vi "ObstacleEnemyRadius.vi"(4 "Goal":dbl[](array[numeric]), 6 "Initial State":dbl[](array[numeric]), 9 "Robot enemy":T1={"id"=0, "function"=enum."Attacker", "x"=0.0, "y"=0.0, "orientation"=0.0, "v_tangent"=0.0, "v_normal"=0.0, "v_ang"=0.0, "kick_x"=0.0, "kick_z"=0.0, "dribble"=FALSE, "Timestamp"=timestamp(0 s since 1904-01-01), "estimatives"={"est_v_tangent"=0.0, "est_v_normal"=0.0, "est_vx"=0.0, "est_vy"=0.0, "Pos Robot Est"=[]}, "dest_x_kick"=0.0, "dest_y_kick"=0.0, "Gap Coord"=[], "States"=enum."GoToTangent", "Path "=[], "Path  Smooth"=[], "Dest"=[]}, 10 "Robot in":T1={"id"=0, "function"=enum."Attacker", "x"=0.0, "y"=0.0, "orientation"=0.0, "v_tangent"=0.0, "v_normal"=0.0, "v_ang"=0.0, "kick_x"=0.0, "kick_z"=0.0, "dribble"=FALSE, "Timestamp"=timestamp(0 s since 1904-01-01), "estimatives"={"est_v_tangent"=0.0, "est_v_normal"=0.0, "est_vx"=0.0, "est_vy"=0.0, "Pos Robot Est"=[]}, "dest_x_kick"=0.0, "dest_y_kick"=0.0, "Gap Coord"=[], "States"=enum."GoToTangent", "Path "=[], "Path  Smooth"=[], "Dest"=[]}) -> (2 "obstacle enemy radius":dbl)   [LabVIEW 2017]
uses:
  Core/AI Robot.ctl
  Intel/Functions Enum.ctl
  Intel/AttackerStates.ctl
  PathDests.ctl
  PathDest.ctl
  <vilib>/Analysis/_algsub.llb/Real Vector Norm.vi
  <vilib>/Analysis/NI_AALPro.lvlib
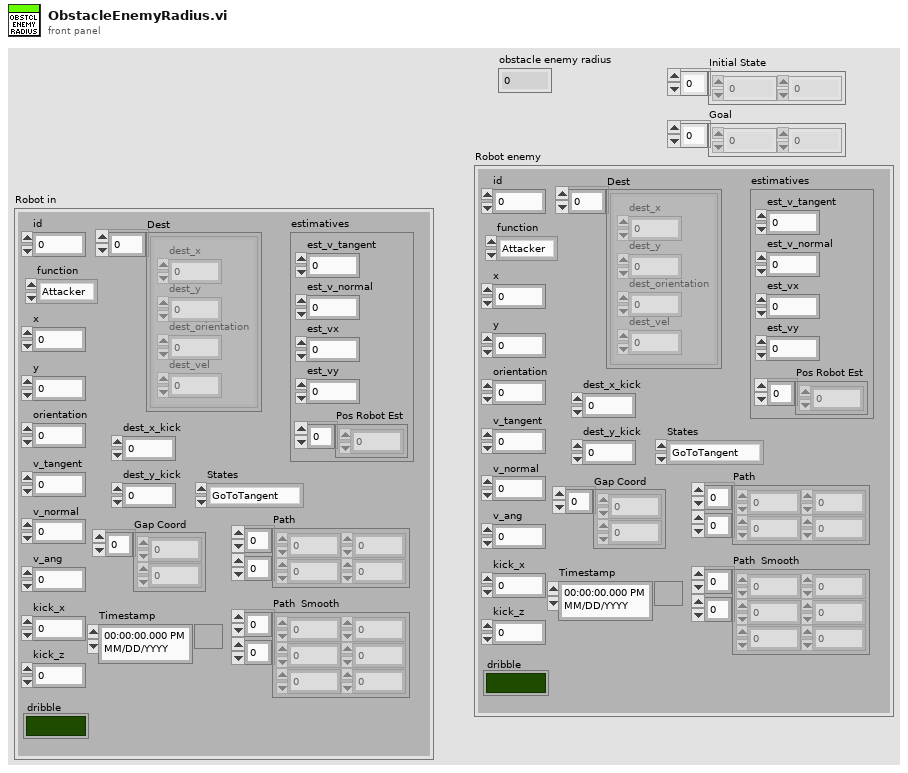
[diagram p1: front panel]
types:
  T1 = typedef "AI Robot.ctl" = cluster{"id":u32, "function":T2, "x":dbl, "y":dbl, "orientation":dbl, "v_tangent":dbl, "v_normal":dbl, "v_ang":dbl, "kick_x":dbl, "kick_z":dbl, "dribble":bool, "Timestamp":timestamp, "estimatives":cluster{"est_v_tangent":dbl, "est_v_normal":dbl, "est_vx":dbl, "est_vy":dbl, "Pos Robot Est":dbl[]}, "dest_x_kick":dbl, "dest_y_kick":dbl, "Gap Coord":dbl[], "States":T3, "Path ":dbl[][], "Path  Smooth":dbl[][], "Dest":T4}
  T2 = typedef "Functions Enum.ctl" = enum16{"Attacker", "Goalie", "Defender", "Striker", "Goto 0", "Dummy", "Kicker", "ZigZag"}
  T3 = typedef "AttackerStates.ctl" = enum16{"Pass", "GoToTangent", "BallGetting", "GoToKick", ""}
  T4 = typedef "PathDests.ctl" = T5[]
  T5 = typedef "PathDest.ctl" = cluster{"dest_x":dbl, "dest_y":dbl, "dest_orientation":dbl, "dest_vel":dbl}
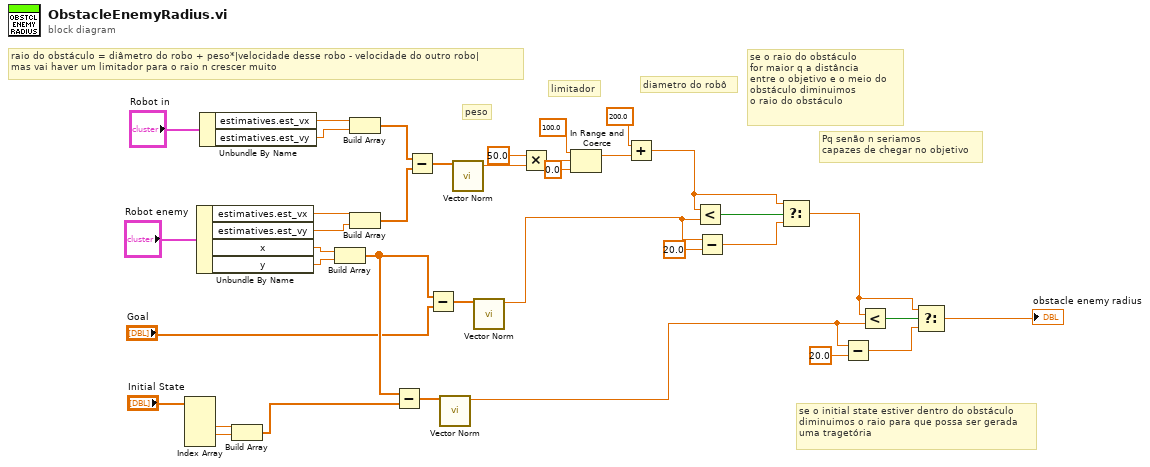
[diagram p0: block diagram]
diagram:
  # "se o initial state estiver dentro do obstáculo\ndiminuimos o raio para que possa ser gerada\numa tragetória"
  # "limitador"
  # "peso"
  # "diametro do robô"
  # "Pq senão n seriamos\ncapazes de chegar no objetivo"
  # "se o raio do obstáculo\nfor maior q a distância \nentre o objetivo e o meio do \nobstáculo diminuimos \no raio do obstáculo"
  # "raio do obstáculo = diâmetro do robo + peso*|velocidade desse robo - velocidade do outro robo|\nmas vai haver um limitador para o raio n crescer muito"
  n1 = Index Array(array="Initial State") -> (element #2=w3:dbl, element #3=w2:dbl)  [unwired: 4 in, 2 out]
  n2 = Unbundle By Name("Robot enemy") -> ("estimatives.est_vx"=w35:dbl, "estimatives.est_vy"=w34:dbl, "x"=w21:dbl, "y"=w20:dbl)
  n3 = Unbundle By Name("Robot in") -> ("estimatives.est_vx"=w33:dbl, "estimatives.est_vy"=w32:dbl)
  n4 = Build Array(w3, w2) -> (w1:dbl[])
  n5 = Build Array(w21, w20) -> (w12:dbl[])
  n6 = Build Array(w33, w32) -> (w31:dbl[])
  n7 = Build Array(w35, w34) -> (w30:dbl[])
  n8 = Subtract(x=w12, y=w1) -> (x-y=w13:dbl[])
  n9 = Subtract(x=w31, y=w30) -> (x-y=w29:dbl[])
  n10 = Subtract(x=w12, y="Goal") -> (x-y=w19:dbl[])
  n11 = call-poly <vilib>:"Vector Norm.vi"("Input Vector"=w13) -> ("norm"=w6:dbl)  [unwired: 9 in, 1 out]
  n12 = call-poly <vilib>:"Vector Norm.vi"("Input Vector"=w29) -> ("norm"=w28:dbl)  [unwired: 9 in, 1 out]
  n13 = call-poly <vilib>:"Vector Norm.vi"("Input Vector"=w19) -> ("norm"=w16:dbl)  [unwired: 9 in, 1 out]
  n14 = Multiply(x=50.0, y=w28) -> (x*y=w26:dbl)
  n15 = In Range and Coerce(upper limit=100.0, x=w26, lower limit=0.0) -> (coerced(x)=w23:dbl)  [unwired: 1 out]
  n16 = Add(x=200.0, y=w23) -> (x+y=w17:dbl)
  n17 = Less?(x=w17, y=w16) -> (x < y?=w18:bool)
  n18 = Subtract(x=w16, y=20.0) -> (x-y=w14:dbl)
  n19 = Select(t=w17, s=w18, f=w14) -> (s? t:f=w8:dbl)
  n20 = Subtract(x=w6, y=20.0) -> (x-y=w5:dbl)
  n21 = Less?(x=w8, y=w6) -> (x < y?=w10:bool)
  n22 = Select(t=w8, s=w10, f=w5) -> (s? t:f=→"obstacle enemy radius":dbl)
